vi "Read Timeout.vi"(8 "error in (no error)":errorcluster, 11 "BaseMessage in":refnum<class "BaseMessage.lvclass">) -> (0 "error out":errorcluster, 2 "Timeout":i32, 3 "BaseMessage out":refnum<class "BaseMessage.lvclass">)   [LabVIEW 2013, in "BaseMessage.lvclass"]
doc: "The maximum time allowed to wait for a responsw for this message.\nIf zero, do not wait at all (don't expect a response)\nIf -1, wait forever"
uses:
  BaseMessage.lvclass
  BaseMessage.lvclass/BaseMessage.ctl
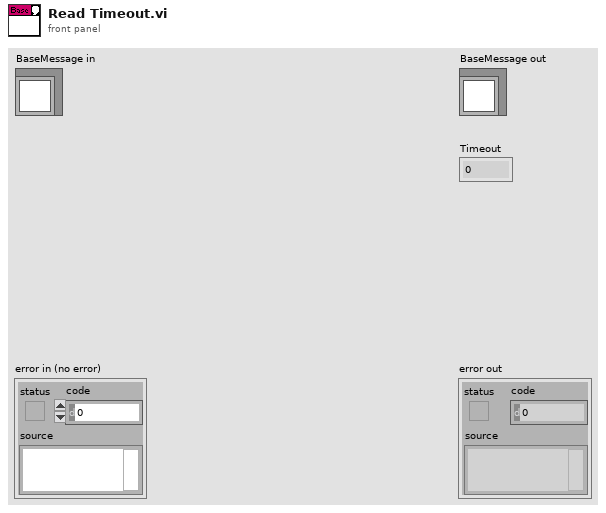
[diagram p1: front panel]
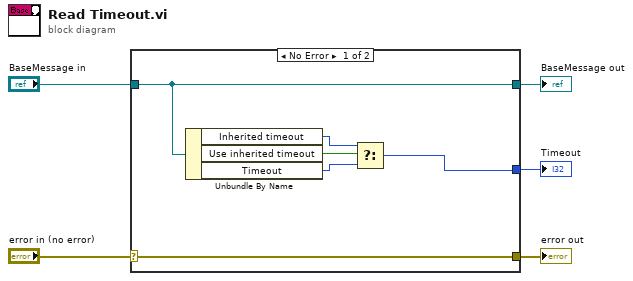
[diagram p0: block diagram]
diagram:
  n1 = case shown="No Error" "error in (no error)" {
    selector: "error in (no error)" -> [w11 w12]
    tunnel: [w11 w12] -> w4
    tunnel: [w10 w13] -> w2
    tunnel: "BaseMessage in" -> [w10 w13]
    tunnel: [w6 _] -> w1
    frame No Error {
      n2 = Unbundle By Name(w10) -> ("Inherited timeout"=w8:i32, "Use inherited timeout"=w9:bool, "Timeout"=w7:i32)
      n3 = Select(t=w8, s=w9, f=w7) -> (s? t:f=w6:i32)
    }
    frame Error {
    }
  }
  "error out" <- w4
  "BaseMessage out" <- w2
  "Timeout" <- w1
